vi "find_close_point_on_side.vi"(9 "ratio_pixel2mil":dbl, 10 "Array":dbl[][](array[numeric]), 11 "fitting clusters":cluster{"fitting array":dbl[][]}[](array[cluster])) -> (2 "D cutting offset array":ext[](array[numeric]), 3 "coord cluster":cluster{dbl[][]}[](array[cluster]))   [LabVIEW 2017]
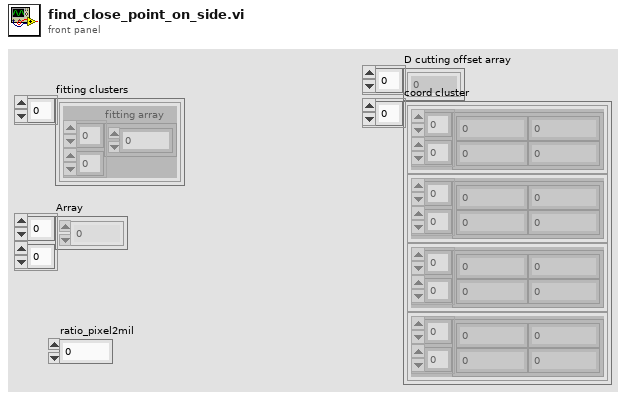
[diagram p1: front panel]
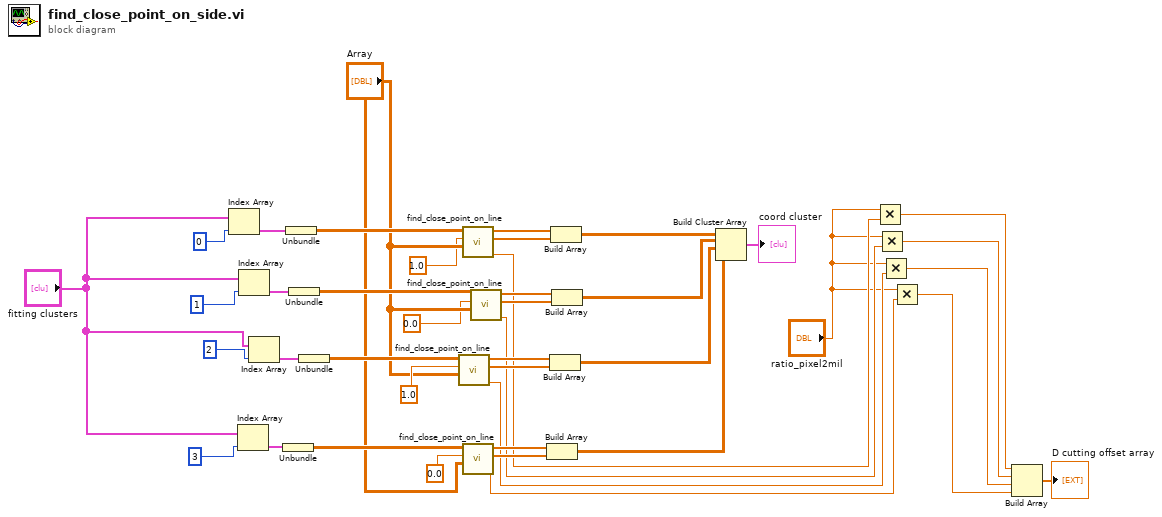
[diagram p0: block diagram]
diagram:
  n1 = Index Array(array="fitting clusters", index=0 ("index (page)")) -> (element=w29:cluster{"fitting array":dbl[][]})
  n2 = Index Array(array="fitting clusters", index=3 ("index (page)")) -> (element=w40:cluster{"fitting array":dbl[][]})
  n3 = Index Array(array="fitting clusters", index=1 ("index (page)")) -> (element=w32:cluster{"fitting array":dbl[][]})
  n4 = Index Array(array="fitting clusters", index=2 ("index (page)")) -> (element=w33:cluster{"fitting array":dbl[][]})
  n5 = Unbundle(w40) -> ("fitting array"=w41:dbl[][])
  n6 = Unbundle(w29) -> ("fitting array"=w36:dbl[][])
  n7 = Unbundle(w32) -> ("fitting array"=w38:dbl[][])
  n8 = Unbundle(w33) -> ("fitting array"=w39:dbl[][])
  n9 = call "find_close_point_on_line.vi"("Array in"="Array", "fitting axis"=1.0, "fitting array"=w39) -> ("d"=w4:ext, "XY online"=w18:dbl[], "XY point"=w19:dbl[])  [unwired: 6 in]
  n10 = call "find_close_point_on_line.vi"("Array in"="Array", "fitting axis"=1.0, "fitting array"=w36) -> ("d"=w9:ext, "XY online"=w22:dbl[], "XY point"=w23:dbl[])  [unwired: 6 in]
  n11 = call "find_close_point_on_line.vi"("Array in"="Array", "fitting axis"=0.0, "fitting array"=w41) -> ("d"=w2:ext, "XY online"=w16:dbl[], "XY point"=w17:dbl[])  [unwired: 6 in]
  n12 = call "find_close_point_on_line.vi"("Array in"="Array", "fitting axis"=0.0, "fitting array"=w38) -> ("d"=w7:ext, "XY online"=w20:dbl[], "XY point"=w21:dbl[])  [unwired: 6 in]
  n13 = Build Array(w17, w16) -> (w12:dbl[][])
  n14 = Build Array(w19, w18) -> (w13:dbl[][])
  n15 = Build Array(w23, w22) -> (w15:dbl[][])
  n16 = Build Array(w21, w20) -> (w14:dbl[][])
  n17 = Build Cluster Array(w15, w14, w13, w12) -> (→"coord cluster":cluster{dbl[][]}[])
  n18 = Multiply(x="ratio_pixel2mil", y=w9) -> (x*y=w8:ext)
  n19 = Multiply(x="ratio_pixel2mil", y=w7) -> (x*y=w6:ext)
  n20 = Multiply(x="ratio_pixel2mil", y=w4) -> (x*y=w5:ext)
  n21 = Multiply(x="ratio_pixel2mil", y=w2) -> (x*y=w1:ext)
  n22 = Build Array(w8, w6, w5, w1) -> (→"D cutting offset array":ext[])
